vi "Evaluate Part 1.vi"() -> ()   [LabVIEW 2021]
uses:
  Proto/Maze.lvclass
panel:
  out "Maze":string[][](array[string])
  out "max value":u64
  in  "Input":string="#.#####################\n#.......#########...###\n#######.#########.#.###\n###.....#.>.>.###.#.###\n###v#####.#v#.###.#.###\n###.>...#.#.#.....#...#\n###v###.#.#.#########.#\n###...#.#.#.......#...#\n#####.#.#.#######.#.###\n#.....#.#.#.......#...#\n#.#####.#.#.#########v#\n#.#...#...#...###...>.#\n#.#.#v#######v###.###v#\n#...#.>.#...>.>.#.###.#\n#####v#.#.###v#.#.###.#\n#.....#...#...#.#.#...#\n#.#########.###.#.#.###\n#...###...#...#...#.###\n###.###.#.###v#####v###\n#...#...#.#.>.>.#.>.###\n#.###.###.#.###.#.#v###\n#.....###...###...#...#\n#####################.#"
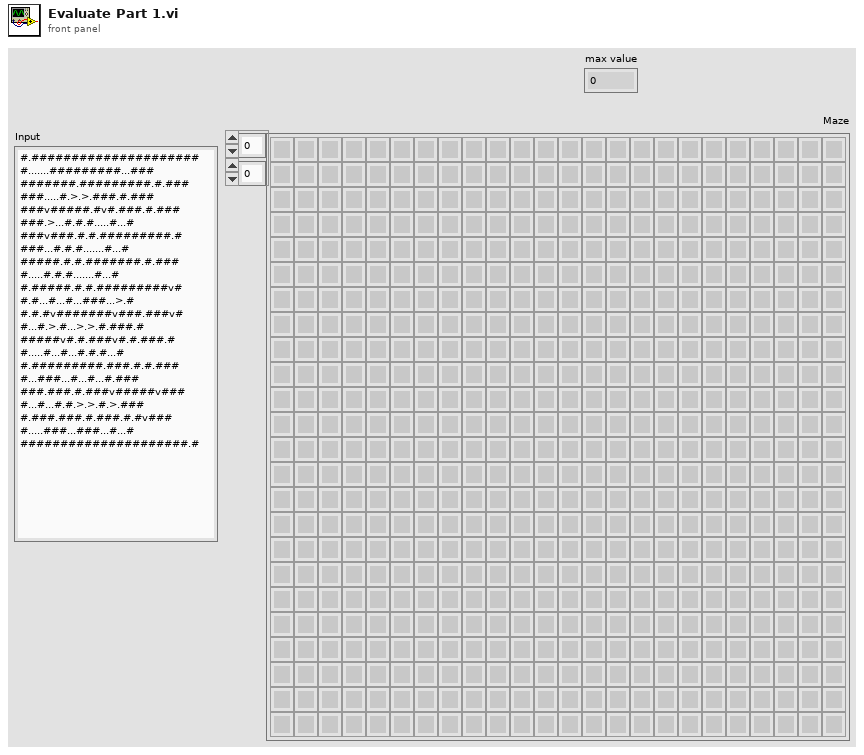
[diagram p1: front panel]
types:
  T1 = cluster{"row":i32, "col":i32, "Arriving from":enum16{"North", "South", "East", "West"}}
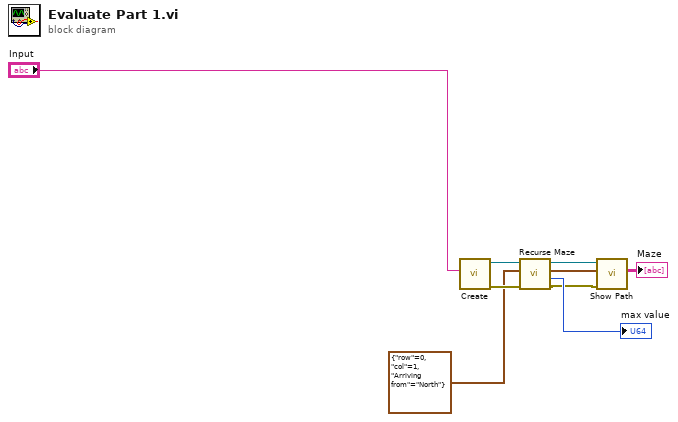
[diagram p0: block diagram]
diagram:
  n1 = call "Create.vi"("Input"="Input") -> ("error out"=w8:errorcluster, "Proto"=w9:refnum<class "Maze.lvclass">)  [unwired: 9 in]
  n2 = call "Recurse Maze.vi"("error in (no error)"=w8, "Current Cell"=T1 {"row"=0, "col"=1, "Arriving from"=enum."North"} ("Possible Steps"), "Maze In"=w9) -> ("error out"=w2:errorcluster, "Step Count"=→"max value":i32, "Steps"=w3:cluster{"row":i32, "col":i32}[], "Maze Out"=w4:refnum<class "Maze.lvclass">)  [unwired: 5 in]
  n3 = call "Show Path.vi"("error in (no error)"=w2, "Steps"=w3, "Maze in"=w4) -> ("Maze"=→"Maze":string[][])  [unwired: 6 in, 2 out]
